vi "calc shooter speed.vi"() -> (0 "Speed":dbl)   [LabVIEW 2011]
uses:
  fg_typedef.ctl
  <vilib>/addons/control/pid/pid.llb/PID Control Input Filter (DBL).vi
  <vilib>/addons/control/pid/NI_PID_pid.lvlib
panel:
  # "Calcualte Shooter Speed based on target height as seen by the robot"
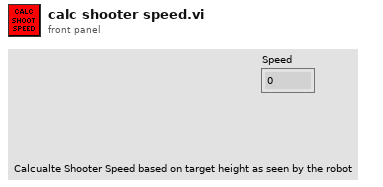
[diagram p1: front panel]
types:
  T1 = typedef "fg_typedef.ctl" = enum16{"Get", "Set"}
  T2 = typedef "vision data.ctl" = cluster{"x":dbl, "y":dbl, "area":dbl, "width":dbl, "height":dbl}
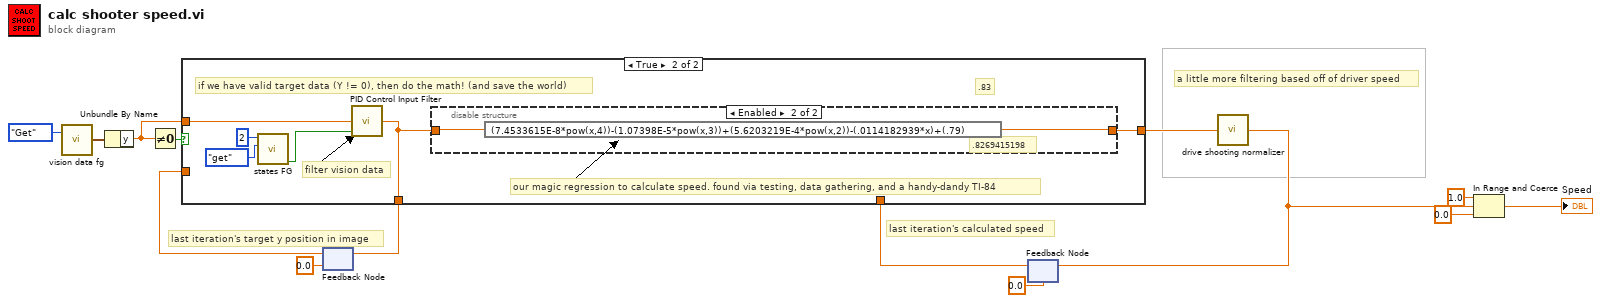
[diagram p0: block diagram]
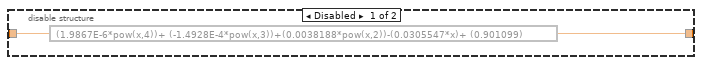
[diagram p3: hidden frame]
diagram:
  # "last iteration's calculated speed"
  # "a little more filtering based off of driver speed"
  # "last iteration's target y position in image"
  n1 = call "vision data fg.vi"("Menu"=fg_typedef."Get") -> ("Data Output"=w13:T2)  [unwired: 1 in]
  n2 = Unbundle By Name(w13) -> ("y"=w11:dbl)
  n3 = Not Equal To 0?(x=w11) -> (x != 0?=w12:bool)
  n4 = feedback #1(0.0 ("output")) -> (w10:dbl)
  n5 = feedback #2(0.0) -> (w3:dbl)
  n6 = case shown="True" w12 {
    tunnel: w11 -> [_ w22]
    tunnel: [w16 w18] -> w4
    tunnel: w10 -> [w16 _]
    tunnel: [w15 w17] -> w2
    tunnel: w3 -> [w15 _]
    frame False {
      # "no good data, keep last values"
    }
    frame True {
      # ".83"
      # "our magic regression to calculate speed. found via testing, data gathering, and a handy-dandy TI-84"
      # "filter vision data"
      # "if we have valid target data (Y != 0), then do the math! (and save the world)"
      n7 = call "states FG.vi"("menu (get)"=enum16{"set", "get"}."get", "Loop ID"=2) -> ("first call?"=w19:bool)  [unwired: 6 in, 3 out]
      n8 = call-poly <vilib>:"PID Control Input Filter.vi"("reinitialize? (F)"=w19, "input"=w22) -> ("output"=w18:dbl)  [unwired: 3 in]
      n9 = disable-structure shown="Enabled" {
        disable-tunnel: w18 -> [w24 w25]
        disable-tunnel: [w23 w26] -> w17
        frame Disabled {
          n10 = expression code="(1.9867E-6*pow(x,4))+ (-1.4928E-4*pow(x,3))+(0.0038188*pow(x,2))-(0.0305547*x)+ (0.901099)"(w24) -> (w23:dbl)
        }
        frame Enabled {
          # ".8269415198"
          n11 = expression code="(7.4533615E-8*pow(x,4))-(1.07398E-5*pow(x,3))+(5.6203219E-4*pow(x,2))-(.0114182939*x)+(.79)"(w25) -> (w26:dbl)
        }
      }
    }
  }
  n12 = feedback-in #1(w4) -> ()
  n13 = call "drive shooting normalizer.vi"("input"=w2) -> ("output"=w1:dbl)
  n14 = feedback-in #2(w1) -> ()
  n15 = In Range and Coerce(upper limit=1.0, x=w1, lower limit=0.0) -> (coerced(x)=→"Speed":dbl)  [unwired: 1 out]
